vi "2 update_mission_queue_TEST.vi"() -> ()   [LabVIEW 2011]
uses:
  2 Typedefs/UTM Location.ctl
  2 Classes/Mission/Mission.lvclass
  2 Classes/MissionQueue/MissionQueue.lvclass
panel:
  in  "Point of Interest 4":T1 {"North" format="%#_10f"; "East" format="%#_8f"}
  in  "Point of Interest 3":T1 {"North" format="%#_10f"; "East" format="%#_8f"}
  in  "Point of Interest 2":T1 {"North" format="%#_10f"; "East" format="%#_8f"}
  in  "Point of Interest":T1 {"North" format="%#_10f"; "East" format="%#_8f"}
  in  "Mission Type":T2(ring)
  # "PoI order for stationkeeping:\nNW, NE, SW, SE"
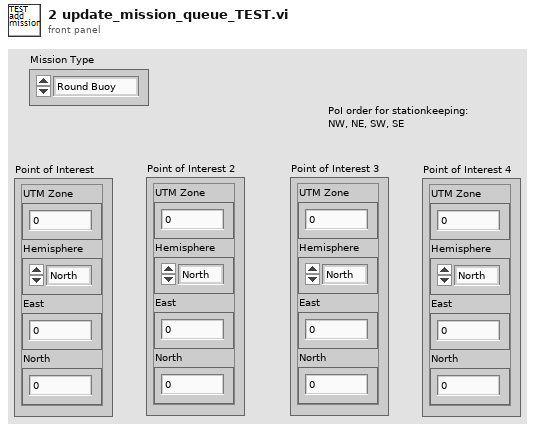
[diagram p1: front panel]
types:
  T1 = typedef "UTM Location.ctl" = cluster{"UTM Zone":dbl, "Hemisphere":enum16{"North", "South"}, "East":dbl, "North":dbl}
  T2 = enum16{"Round Buoy", "Pass Buoys", "Station Keeping"}
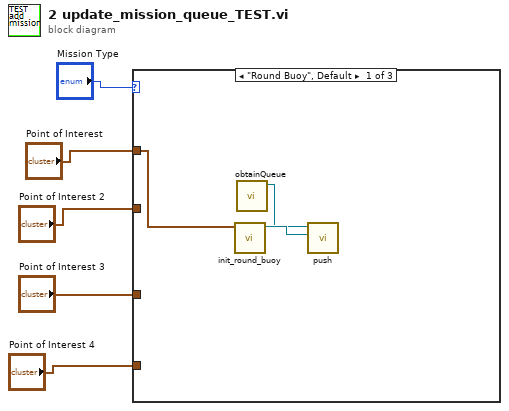
[diagram p0: block diagram]
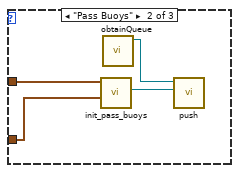
[diagram p2: hidden frame]
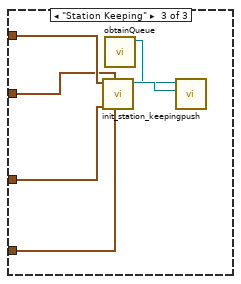
[diagram p3: hidden frame]
diagram:
  n1 = case shown="\"Round Buoy\", Default" "Mission Type" {
    tunnel: "Point of Interest" -> [w6 w10 w16]
    tunnel: "Point of Interest 2" -> [_ w9 w15]
    tunnel: "Point of Interest 4" -> [_ _ w13]
    tunnel: "Point of Interest 3" -> [_ _ w14]
    frame "Round Buoy", Default {
      n2 = call "init_round_buoy.vi"("Buoy to Round"=w6) -> ("Mission out"=w8:refnum<class "Mission.lvclass">)  [unwired: 10 in]
      n3 = call "obtainQueue.vi"() -> ("MissionQueue.lvclass"=w7:refnum<class "MissionQueue.lvclass">)  [unwired: 10 in, 1 out]
      n4 = call "push.vi"("Mission.lvclass"=w8, "MissionQueue in"=w7) -> ()  [unwired: 8 in, 2 out]
    }
    frame "Pass Buoys" {
      n5 = call "init_pass_buoys.vi"("Buoy Pass 2"=w9, "Buoy Pass 1"=w10) -> ("Mission.lvclass"=w12:refnum<class "Mission.lvclass">)  [unwired: 9 in]
      n6 = call "obtainQueue.vi"() -> ("MissionQueue.lvclass"=w11:refnum<class "MissionQueue.lvclass">)  [unwired: 10 in, 1 out]
      n7 = call "push.vi"("Mission.lvclass"=w12, "MissionQueue in"=w11) -> ()  [unwired: 8 in, 2 out]
    }
    frame "Station Keeping" {
      n8 = call "init_station_keeping.vi"("Buoy SE"=w13, "Buoy NE"=w15, "Buoy SW"=w14, "Buoy NW"=w16) -> ("Mission out"=w18:refnum<class "Mission.lvclass">)  [unwired: 7 in]
      n9 = call "obtainQueue.vi"() -> ("MissionQueue.lvclass"=w17:refnum<class "MissionQueue.lvclass">)  [unwired: 10 in, 1 out]
      n10 = call "push.vi"("Mission.lvclass"=w18, "MissionQueue in"=w17) -> ()  [unwired: 8 in, 2 out]
    }
  }
